vi "subHamamatsu_DefineROI.vi"(5 "ROI selection":u16(ring)=11 items=["Full ROI", "Central quad", "Confocal", "", "", "", "", "", "", "patch 1000 width"], 7 "ROI define":bool, 11 "ROI cursor":T1={"Bin"=4, "ROI"={"x offset"=0, "y offset"=0, "x width"=512, "y width"=512}} caption="ROI" {"ROI"."x offset" min=1 max=512 step=1; "ROI"."y offset" min=1 max=512 step=1; "ROI"."x width" min=1 max=512 step=1; "ROI"."y width" min=1 max=512 step=1; "Bin" items=["1x1"=1, "2x2"=2, "4x4"=4]}) -> (3 "ROI out":T1={"Bin"=2, "ROI"={"x offset"=338, "y offset"=256, "x width"=512, "y width"=348}} caption="ROI" {"ROI"."x offset" min=1 max=512 step=1; "ROI"."y offset" min=1 max=512 step=1; "ROI"."x width" min=1 max=512 step=1; "ROI"."y width" min=1 max=512 step=1; "Bin" items=["1x1"=1, "2x2"=2, "4x4"=4]})   [LabVIEW 2015]
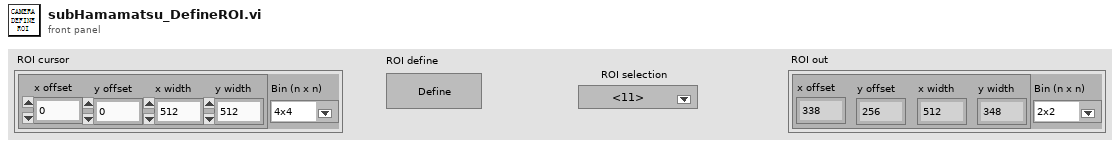
[diagram p1: front panel]
types:
  T1 = cluster{"Bin":u16, "ROI":cluster{"x offset":i32, "y offset":i32, "x width":i32, "y width":i32}}
  T2 = cluster{"x offset":i32, "y offset":i32, "x width":i32, "y width":i32}
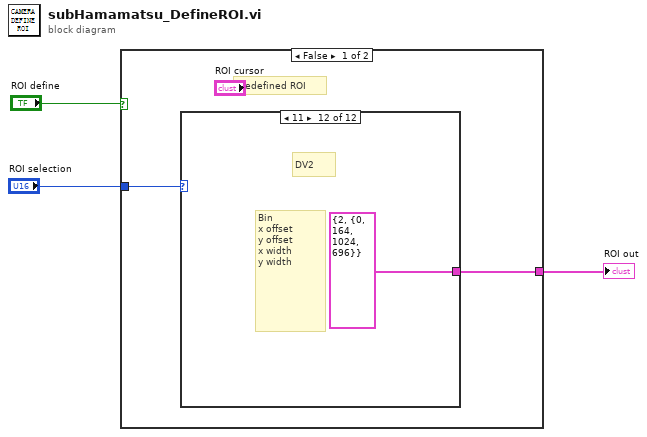
[diagram p0: block diagram]
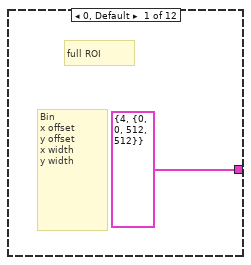
[diagram p2: hidden frame]
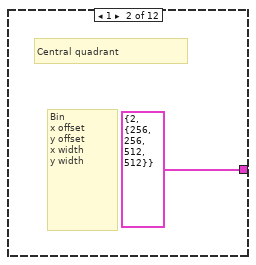
[diagram p3: hidden frame]
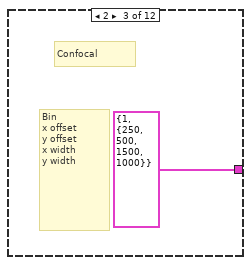
[diagram p4: hidden frame]
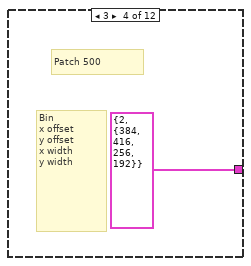
[diagram p5: hidden frame]
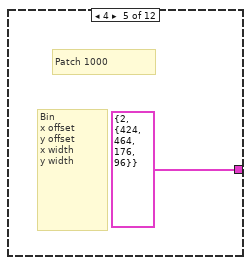
[diagram p6: hidden frame]
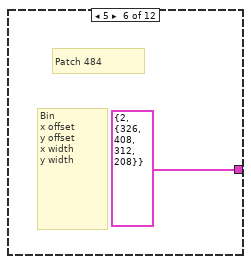
[diagram p7: hidden frame]
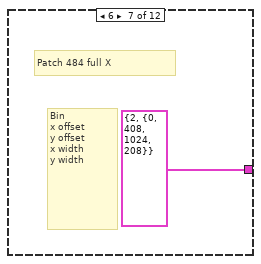
[diagram p8: hidden frame]
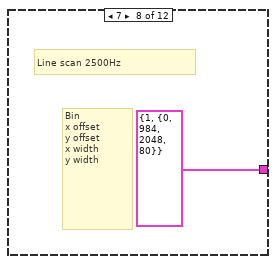
[diagram p9: hidden frame]
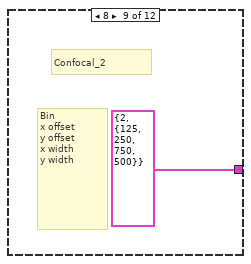
[diagram p10: hidden frame]
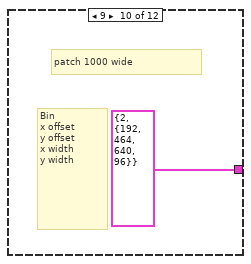
[diagram p11: hidden frame]
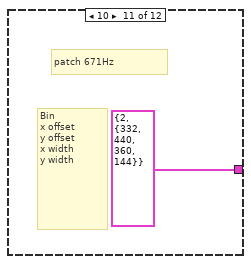
[diagram p12: hidden frame]
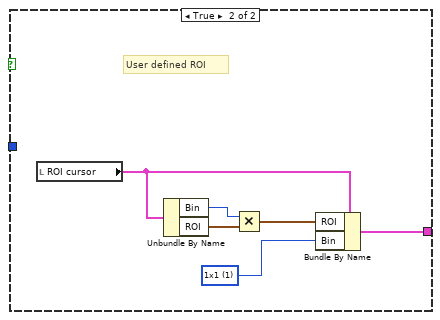
[diagram p13: hidden frame]
diagram:
  n1 = case shown="False" "ROI define" {
    tunnel: [w5 w19] -> w1
    tunnel: "ROI selection" -> [w4 _]
    frame False {
      # "Predefined ROI"
      n2 = case shown="11" w4 {
        tunnel: [T1 {"Bin"=4, "ROI"={"x offset"=0, "y offset"=0, "x width"=512, "y width"=512}} ("ROI cursor 2") T1 {"Bin"=2, "ROI"={"x offset"=256, "y offset"=256, "x width"=512, "y width"=512}} ("ROI cursor 2") T1 {"Bin"=1, "ROI"={"x offset"=250, "y offset"=500, "x width"=1500, "y width"=1000}} ("ROI cursor 2") T1 {"Bin"=2, "ROI"={"x offset"=384, "y offset"=416, "x width"=256, "y width"=192}} ("ROI cursor 2") T1 {"Bin"=2, "ROI"={"x offset"=424, "y offset"=464, "x width"=176, "y width"=96}} ("ROI cursor 2") T1 {"Bin"=2, "ROI"={"x offset"=326, "y offset"=408, "x width"=312, "y width"=208}} ("ROI cursor 2") T1 {"Bin"=2, "ROI"={"x offset"=0, "y offset"=408, "x width"=1024, "y width"=208}} ("ROI cursor 2") T1 {"Bin"=1, "ROI"={"x offset"=0, "y offset"=984, "x width"=2048, "y width"=80}} ("ROI cursor 2") T1 {"Bin"=2, "ROI"={"x offset"=125, "y offset"=250, "x width"=750, "y width"=500}} ("ROI cursor 2") T1 {"Bin"=2, "ROI"={"x offset"=192, "y offset"=464, "x width"=640, "y width"=96}} ("ROI cursor 2") T1 {"Bin"=2, "ROI"={"x offset"=332, "y offset"=440, "x width"=360, "y width"=144}} ("ROI cursor 2") T1 {"Bin"=2, "ROI"={"x offset"=0, "y offset"=164, "x width"=1024, "y width"=696}} ("ROI cursor 2")] -> w5
        frame 0, Default {
          # "Bin\nx offset\ny offset\nx width\ny width"
          # "full ROI"
        }
        frame 1 {
          # "Bin\nx offset\ny offset\nx width\ny width"
          # "Central quadrant"
        }
        frame 2 {
          # "Bin\nx offset\ny offset\nx width\ny width"
          # "Confocal"
        }
        frame 3 {
          # "Bin\nx offset\ny offset\nx width\ny width"
          # "Patch 500"
        }
        frame 4 {
          # "Bin\nx offset\ny offset\nx width\ny width"
          # "Patch 1000"
        }
        frame 5 {
          # "Bin\nx offset\ny offset\nx width\ny width"
          # "Patch 484"
        }
        frame 6 {
          # "Bin\nx offset\ny offset\nx width\ny width"
          # "Patch 484 full X"
        }
        frame 7 {
          # "Bin\nx offset\ny offset\nx width\ny width"
          # "Line scan 2500Hz"
        }
        frame 8 {
          # "Bin\nx offset\ny offset\nx width\ny width"
          # "Confocal_2"
        }
        frame 9 {
          # "Bin\nx offset\ny offset\nx width\ny width"
          # "patch 1000 wide"
        }
        frame 10 {
          # "Bin\nx offset\ny offset\nx width\ny width"
          # "patch 671Hz"
        }
        frame 11 {
          # "Bin\nx offset\ny offset\nx width\ny width"
          # "DV2"
        }
      }
    }
    frame True {
      w18 = u16 1 items=["1x1"=1, "2x2"=2, "4x4"=4] ("Bin (n x n)")
      # "User defined ROI"
      n3 = local read "ROI cursor"() -> (w20:T1)
      n4 = Unbundle By Name(w20) -> ("Bin"=w23:u16, "ROI"=w22:T2)
      n5 = Multiply(x=w23, y=w22) -> (x*y=w21:T2)
      n6 = Bundle By Name(cluster=w20, "ROI"=w21, "Bin"=w18) -> (w19:T1)
    }
  }
  "ROI out" <- w1
